vi "cc_close.vi"(2 "error in (no error)":errorcluster, 3 "VISA In":refnum<visa-resource-name>) -> (0 "error out":errorcluster)   [LabVIEW 2020]
doc: "Closes a connection."
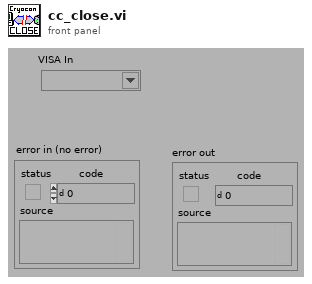
[diagram p1: front panel]
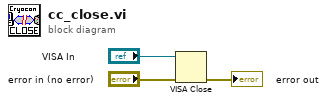
[diagram p0: block diagram]
diagram:
  n1 = VISA Close(VISA resource name="VISA In", error in (no error)="error in (no error)") -> (error out=→"error out":errorcluster)
